vi "Histerisis.vi"() -> ()   [LabVIEW 2020]
uses:
  <vilib>/numeric/Random Number (Range) U64.vi
  <vilib>/numeric/sub_Random U32.vi
panel:
  out "Rango":bool
  out "Histeresis":bool
  in  "Min":dbl
  in  "Max":dbl
  out "Numero":u64
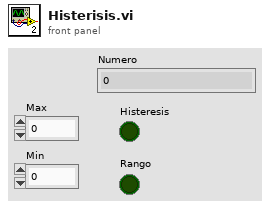
[diagram p1: front panel]
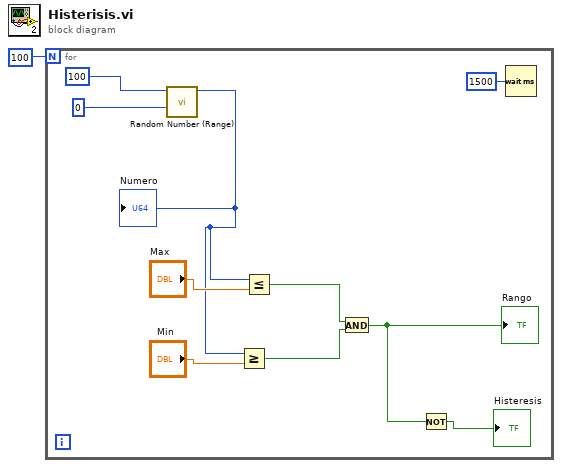
[diagram p0: block diagram]
diagram:
  n1 = for {
    N: 100 -> [_]
    n2 = call-poly <vilib>:"Random Number (Range).vi"("lower bound (0)"=u64 0, "upper bound (100)"=u64 100) -> ("number"=w6:u64)  [unwired: 9 in]
    "Numero" <- w6
    n3 = Greater Or Equal?(x=w6, y="Min") -> (x >= y?=w4:bool)
    n4 = Less Or Equal?(x=w6, y="Max") -> (x <= y?=w5:bool)
    n5 = And(x=w5, y=w4) -> (x .and. y?=w3:bool)
    "Rango" <- w3
    n6 = Not(x=w3) -> (.not. x?=→"Histeresis":bool)
    n7 = Wait (ms)(milliseconds to wait=u32 1500) -> ()  [unwired: 1 out]
  }
